vi "Autotest.vi"(8 "error in (no error)":errorcluster caption="entrée d'erreur (pas d'erreur)", 11 "Class Printer_CAB en entrée":refnum<class "Class Printer_TSC.lvclass">) -> (0 "error out":errorcluster caption="sortie d'erreur", 2 "Autotest Ok ?":bool, 3 "Class Printer_CAB en sortie":refnum<class "Class Printer_TSC.lvclass">)   [LabVIEW 2020, in "Library Instrument & Equipement.lvlib" / "Library Printer.lvlib" / "Class Printer_TSC.lvclass"]
uses:
  Class Printer_TSC.lvclass
  C:/Users/ngarcin/OneDrive - Altyor/Standard TB/Class/Printer/Printer (Default)/Class Printer (Default).lvclass
  Printer (Default)/Class Printer (Default).lvclass
  Class Printer_TSC.lvclass/Class Printer_TSC.ctl
  TSCLIB/TSCLIB.lvlib
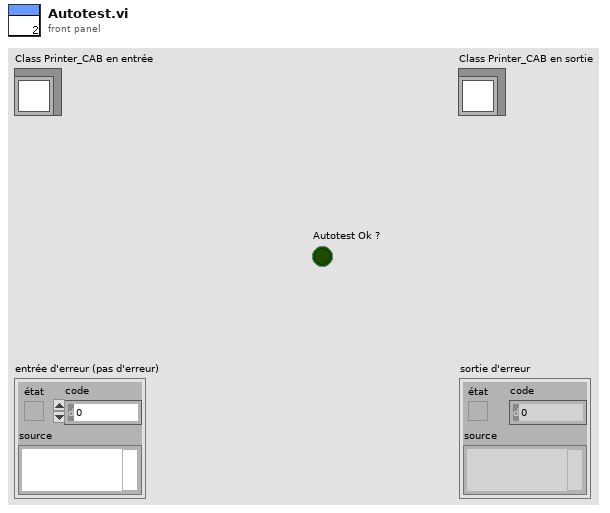
[diagram p1: front panel]
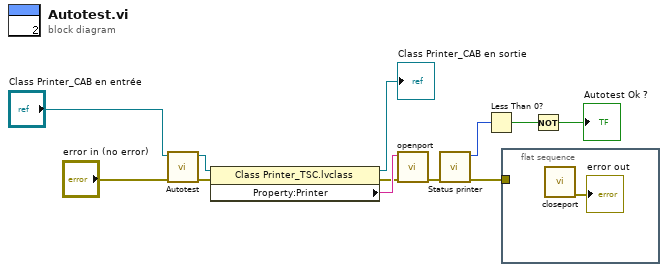
[diagram p0: block diagram]
diagram:
  n1 = call-parent "Autotest.vi"("error in (no error)"="error in (no error)", "Class Printer (Default) en entrée"="Class Printer_CAB en entrée") -> ("error out"=w8:errorcluster, "Class Printer (Default) en sortie"=w10:refnum<class "Class Printer_TSC.lvclass">)  [unwired: 7 in, 1 out]
  n2 = property class="Class Printer_TSC.lvclass"(reference=w10, error in=w8) -> (reference out=→"Class Printer_CAB en sortie":refnum<class "Class Printer_TSC.lvclass">, error out=w6:errorcluster, "Property:Printer"=w7:string)
  n3 = call "openport.vi"("error in (no error)"=w6, "para0"=w7) -> ("error out"=w5:errorcluster)  [unwired: 7 in, 2 out]
  n4 = call "Status printer.vi"("error in (no error)"=w5) -> ("error out"=w1:errorcluster, "function return"=w4:i32)  [unwired: 9 in]
  n5 = Less Than 0?(x=w4) -> (x < 0?=w2:bool)
  n6 = flat-sequence {
    tunnel: w1 -> [_]
    frame #0 {
      n7 = call "closeport.vi"() -> ("error out"=→"error out":errorcluster)  [unwired: 10 in, 1 out]
    }
  }
  n8 = Not(x=w2) -> (.not. x?=→"Autotest Ok ?":bool)
